vi "write test info.vi"(8 "错误输入（无错误）":errorcluster, 9 "测试条件":T2, 10 "粉尘特性":T1, 11 "tdms file in":refnum<k34>) -> (0 "错误输出":errorcluster, 3 "TDMS文件输出":refnum<k34>)   [LabVIEW 2011]
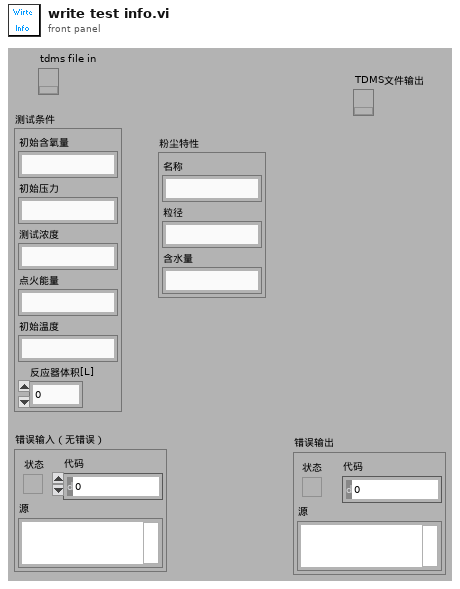
[diagram p1: front panel]
types:
  T1 = typedef "粉尘特性.ctl" = cluster{"名称":string, "粒径":string, "含水量":string}
  T2 = typedef "测试条件.ctl" = cluster{"初始含氧量":string, "初始压力":string, "测试浓度":string, "点火能量":string, "初始温度":string, "反应器体积[L]":dbl}
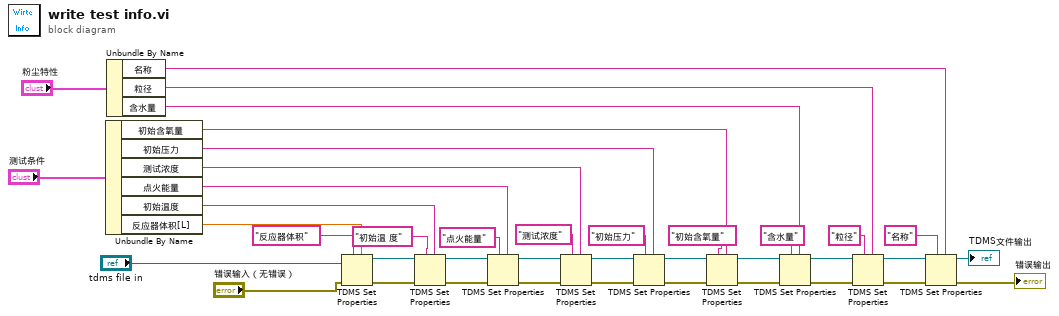
[diagram p0: block diagram]
diagram:
  n1 = Unbundle By Name("测试条件") -> ("初始含氧量"=w22:string, "初始压力"=w23:string, "测试浓度"=w35:string, "点火能量"=w36:string, "初始温度"=w37:string, "反应器体积[L]"=w38:dbl)
  n2 = Unbundle By Name("粉尘特性") -> ("名称"=w20:string, "粒径"=w19:string, "含水量"=w18:string)
  n3 = TDMS Set Properties(5:w38, 7:"反应器体积", 8:"错误输入（无错误）", 11:"tdms file in") -> (0:w28:errorcluster, 3:w17:refnum<k34>)  [unwired: 4 out]
  n4 = TDMS Set Properties(5:w37, 7:"初始温 度", 8:w28, 11:w17) -> (0:w27:errorcluster, 3:w16:refnum<k34>)  [unwired: 4 out]
  n5 = TDMS Set Properties(5:w36, 7:"点火能量", 8:w27, 11:w16) -> (0:w26:errorcluster, 3:w15:refnum<k34>)  [unwired: 4 out]
  n6 = TDMS Set Properties(5:w35, 7:"测试浓度", 8:w26, 11:w15) -> (0:w25:errorcluster, 3:w13:refnum<k34>)  [unwired: 4 out]
  n7 = TDMS Set Properties(5:w23, 7:"初始压力", 8:w25, 11:w13) -> (0:w24:errorcluster, 3:w14:refnum<k34>)  [unwired: 4 out]
  n8 = TDMS Set Properties(5:w22, 7:"初始含氧量", 8:w24, 11:w14) -> (0:w34:errorcluster, 3:w33:refnum<k34>)  [unwired: 4 out]
  n9 = TDMS Set Properties(5:w18, 7:"含水量" ("属性名称"), 8:w34, 11:w33) -> (0:w32:errorcluster, 3:w31:refnum<k34>)  [unwired: 4 out]
  n10 = TDMS Set Properties(5:w19, 7:"粒径" ("属性名称"), 8:w32, 11:w31) -> (0:w30:errorcluster, 3:w29:refnum<k34>)  [unwired: 4 out]
  n11 = TDMS Set Properties(5:w20, 7:"名称" ("属性名称"), 8:w30, 11:w29) -> (0:→"错误输出":errorcluster, 3:→"TDMS文件输出":refnum<k34>)  [unwired: 4 out]
